vi "FGV Init phase.vi"(8 "error in (no error)":errorcluster, 10 "FGV Enum":enum16{"Init", "Check"}(ring)=enum."Check", 11 "Boolean":bool) -> (0 "error out":errorcluster, 3 "Init Completed?":bool)   [LabVIEW 2018, in "Application.lvlib"]
uses:
  Application.lvlib
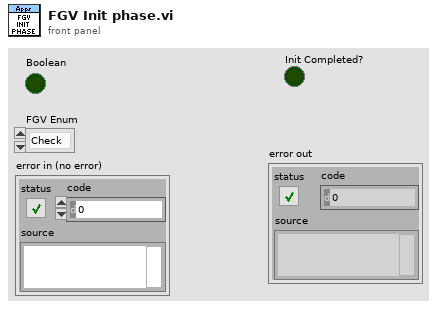
[diagram p1: front panel]
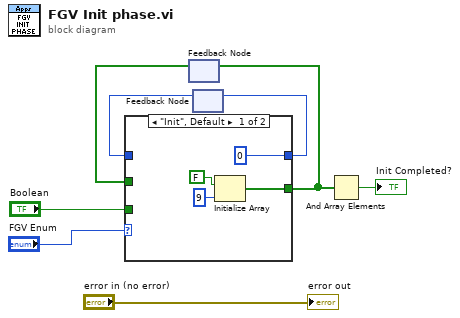
[diagram p0: block diagram]
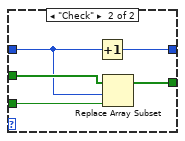
[diagram p2: hidden frame]
diagram:
  n1 = feedback #1() -> (w8:bool[])  [unwired: 1 in]
  n2 = feedback #2() -> (w5:i32)  [unwired: 1 in]
  n3 = case shown="\"Init\", Default" "FGV Enum" {
    tunnel: [w10 w13] -> w4
    tunnel: w8 -> [_ w17]
    tunnel: [0 ("dimension size") w16] -> w6
    tunnel: w5 -> [_ w15]
    tunnel: "Boolean" -> [_ w14]
    frame "Init", Default {
      n4 = Initialize Array(FALSE, 9 ("dimension size")) -> (w10:bool[])
    }
    frame "Check" {
      n5 = Increment(x=w15) -> (x+1=w16:i32)
      n6 = Replace Array Subset(array=w17, new element=w14, index=w15) -> (w13:bool[])
    }
  }
  n7 = feedback-in #1(w4) -> ()
  n8 = feedback-in #2(w6) -> ()
  n9 = And Array Elements(Boolean array=w4) -> (logical AND=→"Init Completed?":bool)
  "error out" <- "error in (no error)"
